vi "Motor PID.vi"(4 "Stop":bool, 7 "output range":cluster{"output high":dbl, "output low":dbl}={"output high"=4000.0, "output low"=-4000.0} {"output low" format="%.2f"; "output high" format="%.2f"}, 8 "dt[s]":dbl=-1.0 format="%.3f", 9 "PID gains":T1={"proportional gain (Kc)"=500.0, "integral time (Ti, min)"=0.001, "derivative time (Td, min)"=0.0} {"derivative time (Td, min)" format="%.3f"; "integral time (Ti, min)" format="%.3f"; "proportional gain (Kc)" format="%.3f"}, 10 "encoder":i32, 11 "vel ref[rps]":dbl) -> (1 "vel actual[rps]":dbl, 2 "pos[rev]":dbl, 3 "duty cycle":i16)   [LabVIEW 2019]
uses:
  <vilib>/addons/control/pid/pid.llb/PID (DBL).vi
  <vilib>/addons/control/pid/NI_PID_pid.lvlib
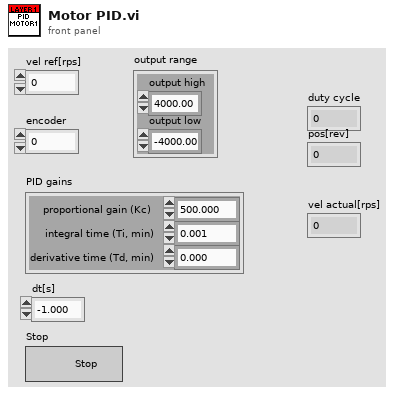
[diagram p1: front panel]
types:
  T1 = cluster{"proportional gain (Kc)":dbl, "integral time (Ti, min)":dbl, "derivative time (Td, min)":dbl}
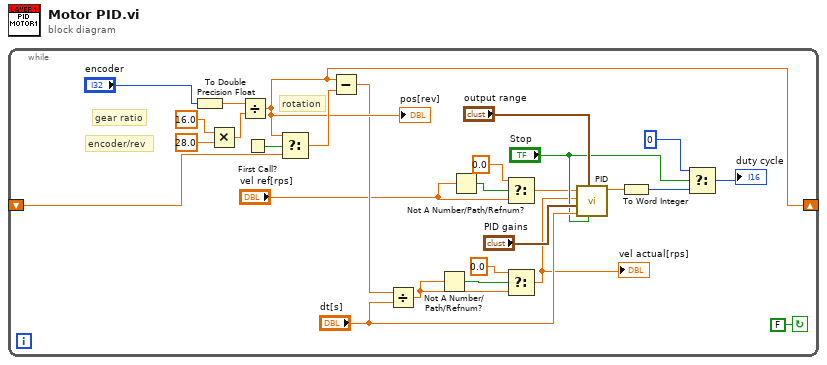
[diagram p0: block diagram]
diagram:
  n1 = while {
    shift-right: [w22] -> _
    shift-left: _ -> [w24]
    stop <- FALSE continue-if-true
    # "rotation"
    # "encoder/rev"
    # "gear ratio"
    n2 = To Double Precision Float(number="encoder") -> (double precision float=w9:dbl)
    n3 = Multiply(x=16.0 ("y"), y=28.0) -> (x*y=w26:dbl)
    n4 = Divide(x=w9, y=w26) -> (x/y=w22:dbl)
    "pos[rev]" <- w22
    n5 = First Call?() -> (First Call?: T/F=w25:bool)
    n6 = Select(t=w22, s=w25, f=w24) -> (s? t:f=w23:dbl)
    n7 = Subtract(x=w22, y=w23) -> (x-y=w21:dbl)
    n8 = Divide(x=w21, y="dt[s]") -> (x/y=w18:dbl)
    n9 = Not A Number/Path/Refnum?(number/path/refnum=w18) -> (NaN/Path/Refnum?=w19:bool)
    n10 = Not A Number/Path/Refnum?(number/path/refnum="vel ref[rps]") -> (NaN/Path/Refnum?=w16:bool)
    n11 = Select(t=0.0, s=w16, f="vel ref[rps]") -> (s? t:f=w7:dbl)
    n12 = Select(t=0.0, s=w19, f=w18) -> (s? t:f=w10:dbl)
    "vel actual[rps]" <- w10
    n13 = call-poly <vilib>:"PID.vi"("reinitialize? (F)"="Stop", "output range"="output range", "dt (s)"="dt[s]", "PID gains"="PID gains", "process variable"=w10, "setpoint"=w7) -> ("output"=w27:dbl)  [unwired: 4 in, 1 out]
    n14 = To Word Integer(number=w27) -> (16bit integer=w8:i16)
    n15 = Select(t=i16 0, s="Stop", f=w8) -> (s? t:f=→"duty cycle":i16)
  }
